vi "QAM Symbol to Waveform.vi"(3 "Symbol Rate (Hz)":dbl=1.0 min=1.0, 4 "Samples / Symbol":i32=1 min=1, 5 "Symbol Listing":cdb[](array[numeric])) -> (0 "sampling info":cluster{"Fs":dbl, "#s":dbl}={"Fs"=1000.0, "#s"=1000.0} {"Fs" format="%.2p"}, 1 "Waveform":waveform(cdb), 2 "output complex waveform":T1 {"Y" format="%.3f"; "dt" format="%^.2e"; "t0" format="%.4f"})   [LabVIEW 2018]
doc: "Converts QAM Symbol listing into waveform with padded sampling"
uses:
  <vilib>/addons/Modulation/Analog/controls/Complex Data Waveform.ctl
  <vilib>/Analysis/2dsp.llb/Upsample (CDB).vi
  <vilib>/Analysis/NI_AALPro.lvlib
  <vilib>/addons/Modulation/niAMT.lvlib
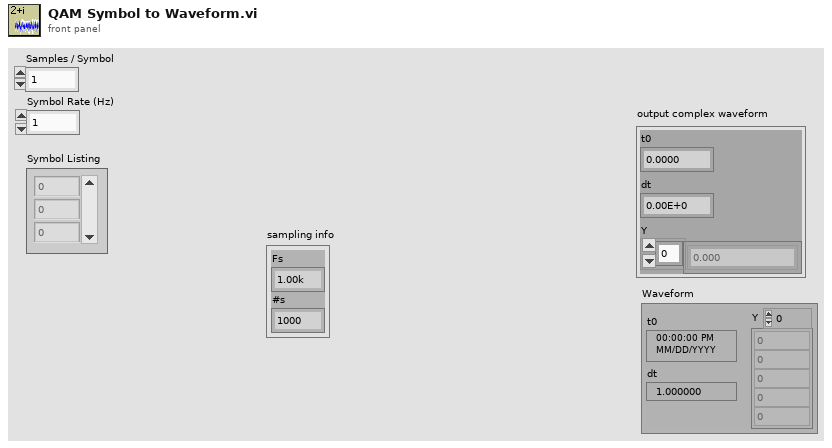
[diagram p1: front panel]
types:
  T1 = typedef "niAMT.lvlib/Complex Data Waveform.ctl" = cluster{"t0":dbl, "dt":dbl, "Y":cdb[]}
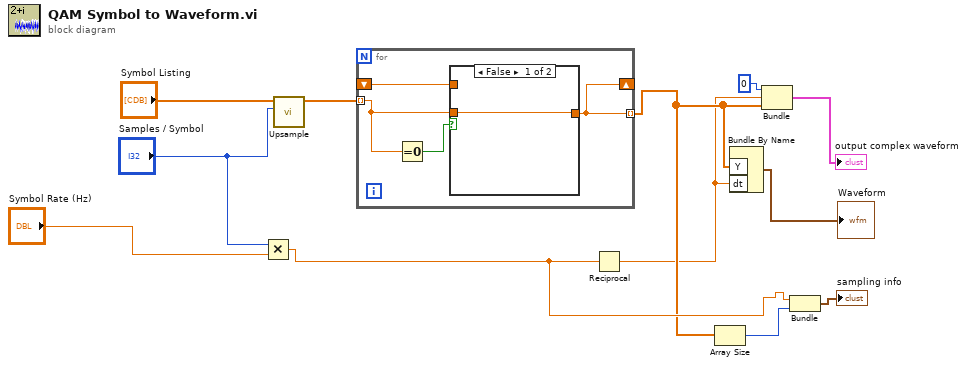
[diagram p0: block diagram]
diagram:
  n1 = Multiply(x="Samples / Symbol", y="Symbol Rate (Hz)") -> (x*y=w8:dbl)
  n2 = call-poly <vilib>:"Upsample.vi"("upsampling factor"="Samples / Symbol", "X"="Symbol Listing") -> ("Upsampled Array"=w11:cdb[])  [unwired: 8 in, 1 out]
  n3 = for {
    tunnel: w11 -> [w15] mode=indexing
    shift-right: [w13] -> _
    shift-left: _ -> [w14]
    tunnel: [w13] -> w4 mode=indexing
    n4 = Equal To 0?(x=w15) -> (x = 0?=w16:bool)
    n5 = case shown="False" w16 {
      tunnel: [w17 w18] -> w13
      tunnel: w15 -> [w17 _]
      tunnel: w14 -> [_ w18]
      frame False {
      }
      frame True {
      }
    }
  }
  n6 = Reciprocal(x=w8) -> (1/x=w3:dbl)
  n7 = Array Size(array=w4) -> (size(s)=w7:i32)
  n8 = Bundle By Name("Y"=w4, "dt"=w3) -> (→"Waveform":waveform(cdb))  [unwired: 1 in]
  n9 = Bundle(0, w3, w4) -> (→"output complex waveform":cluster{i32, dbl, cdb[]})  [unwired: 1 in]
  n10 = Bundle(w8, w7) -> (→"sampling info":cluster{dbl, i32})  [unwired: 1 in]
